vi "Set ROI.vi"(0 "Notifier Name":string, 7 "Camera ROI":T1, 11 "Error In":errorcluster) -> (4 "Notifier Name DUP":string, 15 "Error Out":errorcluster)   [LabVIEW 2020]
uses:
  Camera Controls/Generic Camera ROI.ctl
  Hardware Configuration/Hardware Configuration Controls/Company.ctl
  Hamamatsu/Orca Flash/Orca Flash Controls/Orca Flash ROI.ctl
  Hamamatsu/Orca Flash/Orca Flash Controls/Orca Flash Actions.ctl
  IDS/IDS Controls/IDS Actions.ctl
  IDS/IDS Controls/IDS ROI.ctl
  Photometrics/Prime BSI/R Cubed SITK/Prime BSI R3 Controls/Prime R3 Actions.ctl
  Photometrics/Prime BSI/R Cubed SITK/Prime BSI R3 Controls/Prime R3 ROI.ctl
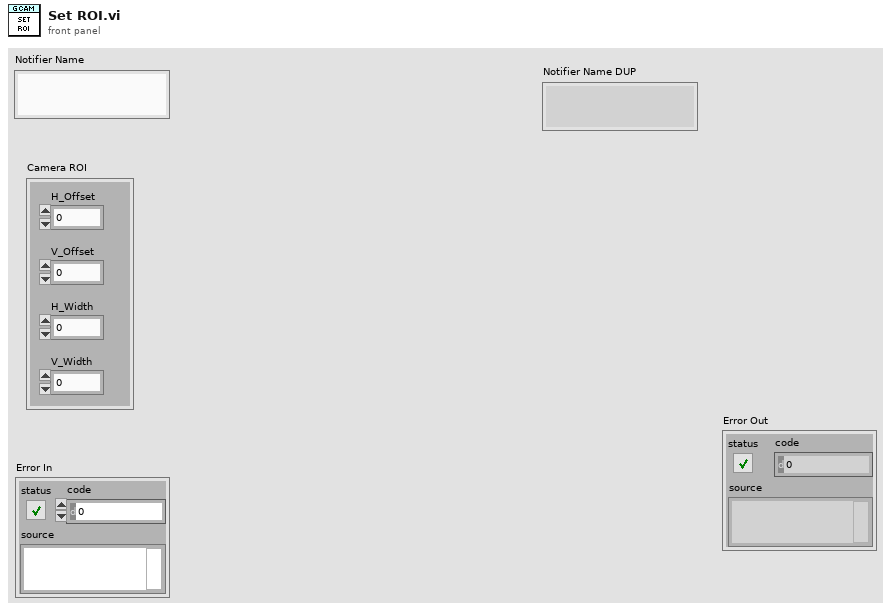
[diagram p1: front panel]
types:
  T1 = typedef "Generic Camera ROI.ctl" = cluster{"H_Offset":u16, "V_Offset":u16, "H_Width":u16, "V_Width":u16}
  T2 = typedef "Company.ctl" = enum16{"AA Opto Electronic", "ASI", "Coherent", "Creset Optics", "CVI", "DAQmx", "Hamamatsu", "IDS", "Mad City Labs", "Marzhauser", "Measurement Computing", "MPB Com", "Olympus", "Photometrics", "PI", "Prior", "Thorlabs"}
  T3 = typedef "Orca Flash Actions.ctl" = enum16{"Idle", "Preview", "Record", "Record Settings", "Set Param", "Get Param", "Set ROI", "Get ROI", "Trigger Source", "Trigger Type", "Progessive Mode", "Area Mode", "Status", "Quit"}
  T4 = typedef "Orca Flash ROI.ctl" = cluster{"H Offset":i32, "V Offset":i32, "H Width":i32, "V Width":i32}
  T5 = typedef "IDS ROI.ctl" = cluster{"H Offset":i32, "V Offset":i32, "H Width":i32, "V Width":i32}
  T6 = typedef "IDS Actions.ctl" = enum16{"Error Check", "Initialize", "Preview", "Record", "Abort", "Record Settings", "Set Parameter", "Get Parameter", "Set ROI", "Get ROI", "Status", "Quit"}
  T7 = typedef "Prime R3 ROI.ctl" = cluster{"X Start":u32, "X End":u32, "X Bin":u32, "Y Start":u32, "Y End":u32, "Y Bin":u32}
  T8 = typedef "Prime R3 Actions.ctl" = enum16{"Error Check", "Initialize", "Preview", "Record", "Abort", "Record Settings", "Set Parameter", "Get Parameter", "Set ROI", "Get ROI", "Status", "Set Trigger", "Quit"}
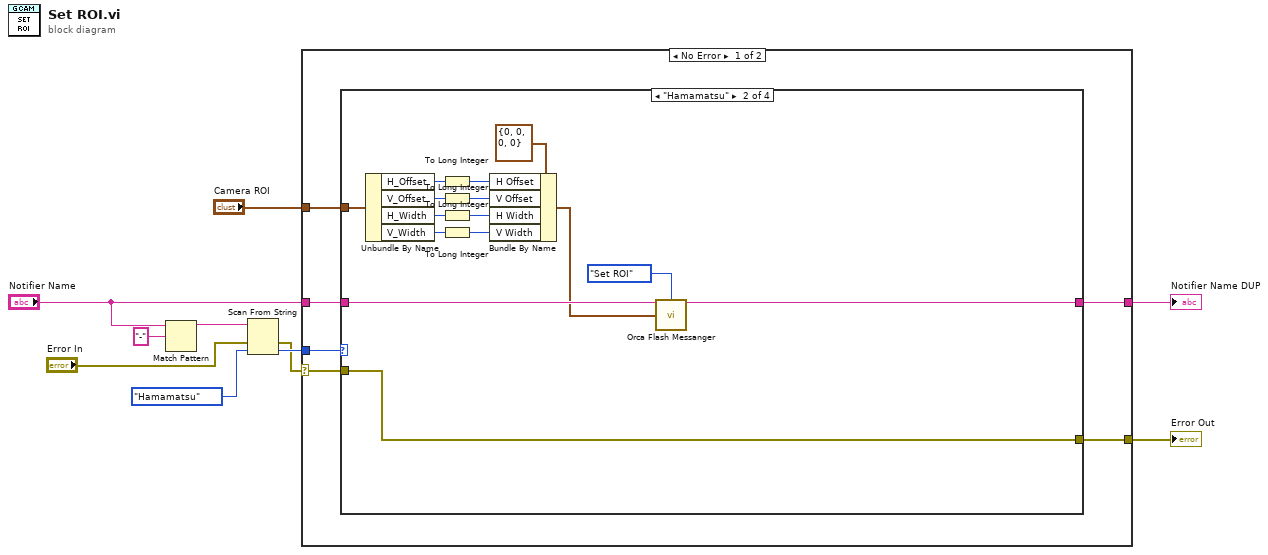
[diagram p0: block diagram]
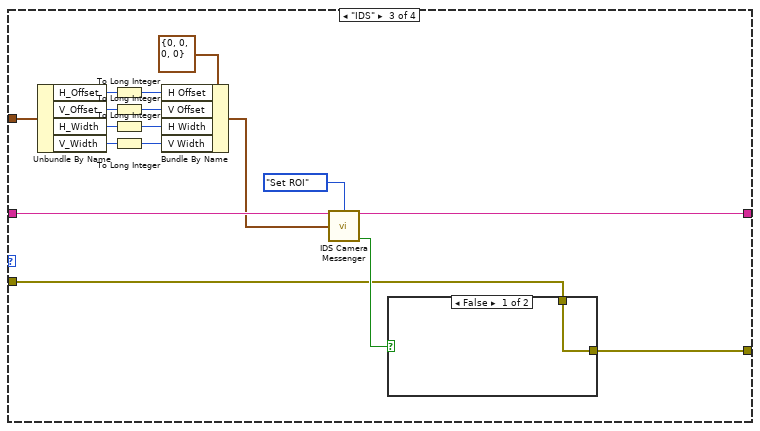
[diagram p3: hidden frame]
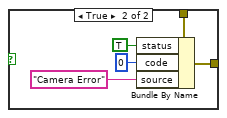
[diagram p4: hidden frame]
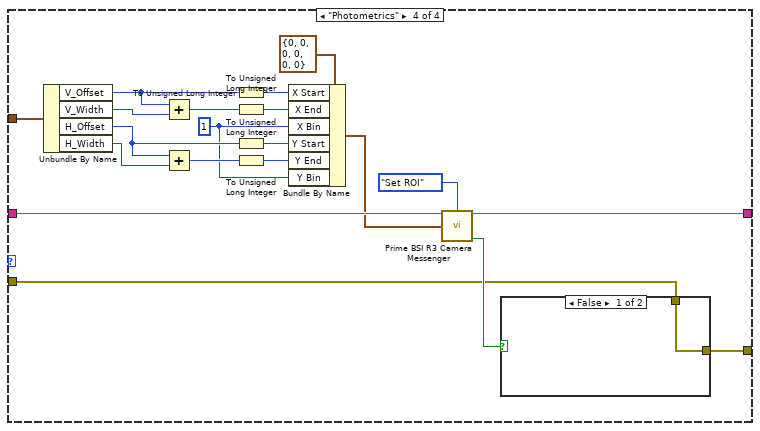
[diagram p5: hidden frame]
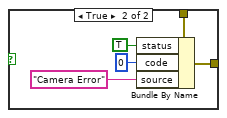
[diagram p6: hidden frame]
diagram:
  n1 = Match Pattern(string="Notifier Name", regular expression="-") -> (before substring=w8:string)  [unwired: 1 in, 3 out]
  n2 = Scan From String(input string=w8, error in="Error In", default 1=Company."Hamamatsu" ("Company")) -> (error out=w4:errorcluster, output 1=w7:T2)  [unwired: 2 in, 2 out]
  n3 = case shown="No Error" w4 {
    selector: w4 -> [w14 w83]
    tunnel: w7 -> [w16 _]
    tunnel: "Notifier Name" -> [w15 w84]
    tunnel: [w13 w84] -> w3
    tunnel: [w12 w83] -> w2
    tunnel: "Camera ROI" -> [w11 _]
    frame No Error {
      n4 = case shown="\"Hamamatsu\"" w16 {
        tunnel: w15 -> [w18 w33 w50 w76]
        tunnel: w14 -> [w17 w31 w46 w73]
        tunnel: [w18 w32 w49 w75] -> w13
        tunnel: [w17 w31 w45 w72] -> w12
        tunnel: w11 -> [_ w21 w35 w58]
        frame Default {
        }
        frame "Hamamatsu" {
          n5 = Unbundle By Name(w21) -> ("H_Offset"=w26:u16, "V_Offset"=w27:u16, "H_Width"=w28:u16, "V_Width"=w29:u16)
          n6 = To Long Integer(number=w26) -> (32bit integer=w25:i32)
          n7 = To Long Integer(number=w27) -> (32bit integer=w24:i32)
          n8 = To Long Integer(number=w28) -> (32bit integer=w23:i32)
          n9 = To Long Integer(number=w29) -> (32bit integer=w22:i32)
          n10 = Bundle By Name(cluster=T4 {"H Offset"=0, "V Offset"=0, "H Width"=0, "V Width"=0} ("sCMOS ROI"), "H Offset"=w25, "V Offset"=w24, "H Width"=w23, "V Width"=w22) -> (w20:T4)
          n11 = call "Orca Flash Messanger.vi"("Notifier Name"=w33, "Camera Actions"=Orca_Flash_Actions."Set ROI", "sCMOS ROI"=w20) -> ("Notifier Name Dup"=w32:string)  [unwired: 8 in, 4 out]
        }
        frame "IDS" {
          n12 = Unbundle By Name(w35) -> ("H_Offset"=w40:u16, "V_Offset"=w41:u16, "H_Width"=w42:u16, "V_Width"=w43:u16)
          n13 = To Long Integer(number=w40) -> (32bit integer=w39:i32)
          n14 = To Long Integer(number=w41) -> (32bit integer=w38:i32)
          n15 = To Long Integer(number=w42) -> (32bit integer=w37:i32)
          n16 = To Long Integer(number=w43) -> (32bit integer=w36:i32)
          n17 = Bundle By Name(cluster=T5 {"H Offset"=0, "V Offset"=0, "H Width"=0, "V Width"=0} ("sCMOS ROI"), "H Offset"=w39, "V Offset"=w38, "H Width"=w37, "V Width"=w36) -> (w34:T5)
          n18 = call "IDS Camera Messenger.vi"("Notifier Name"=w50, "IDS Actions"=IDS_Actions."Set ROI", "ROI Setup"=w34) -> ("Notifier Name (Dup)"=w49:string, "Error?"=w47:bool)  [unwired: 7 in, 4 out]
          n19 = case shown="False" w47 {
            tunnel: w46 -> [w51 w56]
            tunnel: [w51 w55] -> w45
            frame False {
            }
            frame True {
              n20 = Bundle By Name(cluster=w56, "status"=TRUE, "code"=0, "source"="Camera Error") -> (w55:errorcluster)
            }
          }
        }
        frame "Photometrics" {
          w61 = u32 1 ("number")
          n21 = Unbundle By Name(w58) -> ("V_Offset"=w69:u16, "V_Width"=w67:u16, "H_Offset"=w63:u16, "H_Width"=w62:u16)
          n22 = Add(x=w69, y=w67) -> (x+y=w68:u16)
          n23 = Add(x=w63, y=w62) -> (x+y=w65:u16)
          n24 = To Unsigned Long Integer(number=w69) -> (unsigned 32bit integer=w70:u32)
          n25 = To Unsigned Long Integer(number=w68) -> (unsigned 32bit integer=w60:u32)
          n26 = To Unsigned Long Integer(number=w63) -> (unsigned 32bit integer=w64:u32)
          n27 = To Unsigned Long Integer(number=w65) -> (unsigned 32bit integer=w66:u32)
          n28 = Bundle By Name(cluster=T7 {"X Start"=0, "X End"=0, "X Bin"=0, "Y Start"=0, "Y End"=0, "Y Bin"=0} ("sCMOS ROI"), "X Start"=w70, "X End"=w60, "X Bin"=w61, "Y Start"=w64, "Y End"=w66, "Y Bin"=w61) -> (w57:T7)
          n29 = call "Prime BSI R3 Camera Messenger.vi"("Notifier Name"=w76, "Prime Actions"=Prime_R3_Actions."Set ROI", "ROI Setup"=w57) -> ("Notifier Name (Dup)"=w75:string, "Error?"=w74:bool)  [unwired: 7 in, 4 out]
          n30 = case shown="False" w74 {
            tunnel: w73 -> [w77 w82]
            tunnel: [w77 w81] -> w72
            frame False {
            }
            frame True {
              n31 = Bundle By Name(cluster=w82, "status"=TRUE, "code"=0, "source"="Camera Error") -> (w81:errorcluster)
            }
          }
        }
      }
    }
    frame Error {
    }
  }
  "Error Out" <- w2
  "Notifier Name DUP" <- w3
